vi "LVAPT-GIT-LeaveDailyBranch.vi"(11 "path":path) -> ()   [LabVIEW 2019]
uses:
  <vilib>/Hampel Software Engineering/Git API/Git API/GIT-api.lvclass/GIT-api.ctl
  <vilib>/Hampel Software Engineering/Git API/Git API/Accessors/GIT-Set Working Dir.vi
  <vilib>/Hampel Software Engineering/Git API/Git API/GIT-api.lvclass
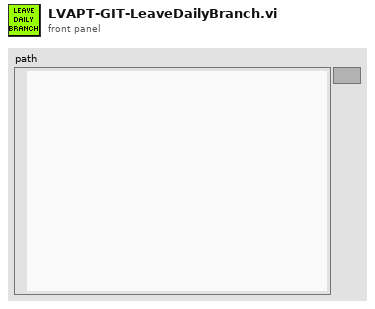
[diagram p1: front panel]
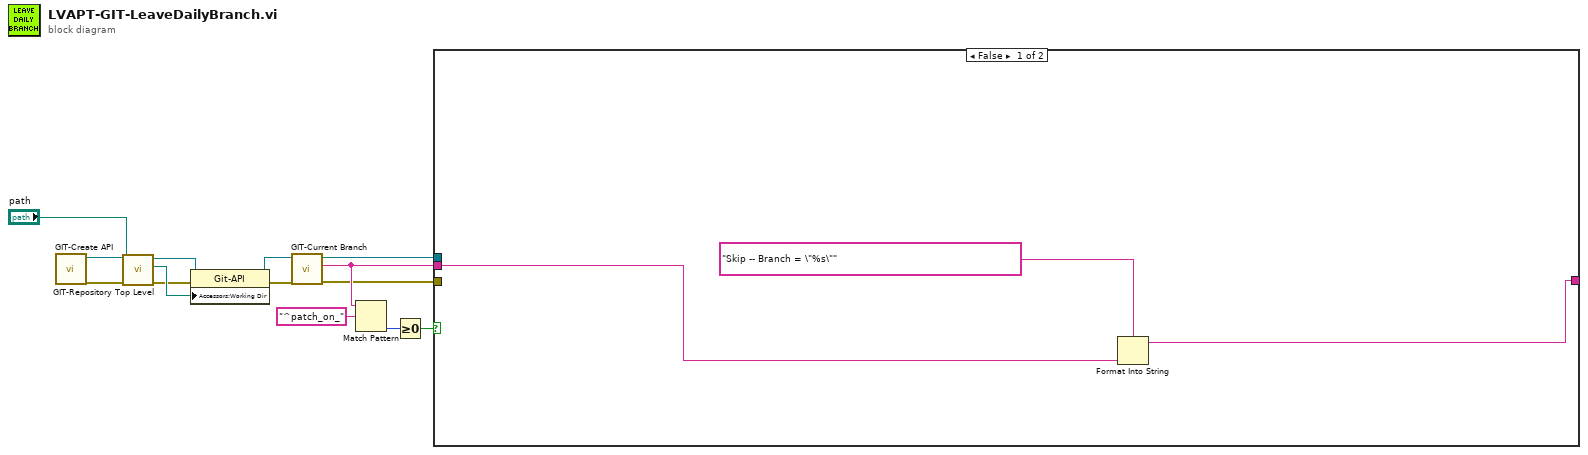
[diagram p0: block diagram]
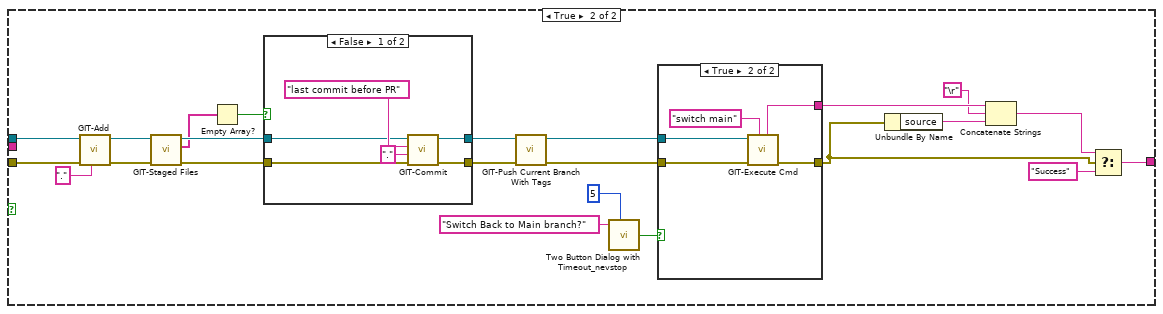
[diagram p2: hidden frame]
diagram:
  n1 = call <vilib>:"GIT-Create API.vi"() -> ("error out"=w7:errorcluster, "git-api out"=w6:refnum<class "GIT-api.lvclass">)  [unwired: 10 in]
  n2 = call <vilib>:"GIT-Repository Top Level.vi"("error in"=w7, "Current Path"="path", "git-api in"=w6) -> ("error out"=w1:errorcluster, "Repo Top Level Path"=w3:path, "git-api out"=w2:refnum<class "GIT-api.lvclass">)  [unwired: 6 in]
  n3 = property class="Git-API"(reference=w2, error in=w1, "Accessors:Working Dir"=w3) -> (reference out=w4:refnum<class "GIT-api.lvclass">, error out=w5:errorcluster)
  n4 = call <vilib>:"GIT-Current Branch.vi"("error in"=w5, "git-api in"=w4) -> ("error out"=w8:errorcluster, "current branch"=w13:string, "git-api out"=w9:refnum<class "GIT-api.lvclass">)  [unwired: 7 in]
  n5 = Match Pattern(string=w13, regular expression="^patch_on_") -> (offset past match=w11:i32)  [unwired: 1 in, 3 out]
  n6 = Greater Or Equal To 0?(x=w11) -> (x >= 0?=w12:bool)
  n7 = case shown="False" w12 {
    tunnel: w8 -> [_ w36]
    tunnel: w9 -> [_ w35]
    tunnel: w13 -> [w17 _]
    tunnel: [w15 w18] -> _
    frame False {
      n8 = Format Into String(format string="Skip -- Branch = \"%s\"" ("f"), w17) -> (resulting string=w15:string)  [unwired: 2 in, 1 out]
    }
    frame True {
      n9 = call <vilib>:"GIT-Add.vi"("param"=".", "error in"=w36, "git-api in"=w35) -> ("error out"=w28:errorcluster, "git-api out"=w30:refnum<class "GIT-api.lvclass">)  [unwired: 6 in, 1 out]
      n10 = call <vilib>:"GIT-Staged Files.vi"("error in"=w28, "Git-API in"=w30) -> ("error out"=w27:errorcluster, "Staged Files"=w26:string[], "Git-API out"=w29:refnum<class "GIT-api.lvclass">)  [unwired: 7 in]
      n11 = Empty Array?(array=w26) -> (empty?=w25:bool)
      n12 = case shown="False" w25 {
        tunnel: [w45 w48] -> w40
        tunnel: [w44 w47] -> w38
        tunnel: w29 -> [w42 w48]
        tunnel: w27 -> [w41 w47]
        frame False {
          n13 = call <vilib>:"GIT-Commit.vi"("error in"=w41, "params"=".", "msg"="last commit before PR", "Git-API in"=w42) -> ("error out"=w44:errorcluster, "Git-API out"=w45:refnum<class "GIT-api.lvclass">)  [unwired: 6 in]
        }
        frame True {
        }
      }
      n14 = call <vilib>:"GIT-Push Current Branch With Tags.vi"("error in"=w38, "Git-API in"=w40) -> ("error out"=w37:errorcluster, "Git-API out"=w39:refnum<class "GIT-api.lvclass">)  [unwired: 8 in]
      n15 = call <userlib>:"Two Button Dialog with Timeout_nevstop.vi"("message"="Switch Back to Main branch?", "T Timeout(-1 s)"=5) -> ("T button?"=w32:bool)  [unwired: 3 in]
      n16 = case shown="True" w32 {
        tunnel: [w49 w54] -> w20
        tunnel: [_ w53] -> w22
        tunnel: w39 -> [_ w51]
        tunnel: w37 -> [w49 w50]
        frame False {
        }
        frame True {
          n17 = call <vilib>:"GIT-Execute Cmd.vi"("Command"="switch main" ("format string"), "error in"=w50, "Git-API in"=w51) -> ("error out"=w54:errorcluster, "std out"=w53:string)  [unwired: 6 in, 1 out]
        }
      }
      n18 = Unbundle By Name(w20) -> ("source"=w23:string)
      n19 = Concatenate Strings(w22, "\r", w23) -> (w24:string)
      n20 = Select(t=w24, s=w20, f="Success") -> (s? t:f=w18:string)
    }
  }
